vi "Teleop.vi"(10 "Match Info":T3={"Autonomous Elapsed Seconds"=0.0, "TeleOp Elapsed Seconds"=0.0, "Disabled Elapsed Seconds"=0.0, "Visited Autonomous"=FALSE, "Visited TeleOp"=FALSE, "Visited Disabled"=FALSE, "Autonomous Settings"={"Autonomous Style"=enum."Independent", "VI Refnum"=refnum}}, 11 "Call Context":T4) -> ()   [LabVIEW 2020]
doc: "This VI is called for each TeleOp packet received from the DS where the robot is not disabled. It is often used to read from the joysticks and update I/O or to update setpoints for timed control loops. It should complete and return within 20 milliseconds or it may miss DS packets."
uses:
  <vilib>/Rock Robotics/WPI/ThirdParty/Phoenix-LabVIEW/Motor Controller/Controls/CTRE_Phoenix_MotorControl_ControlMode.ctl
  TitanLib/Lib/TitanLib.lvlib
  TitanLib/Lib/Piston Hold.vi
  <vilib>/Rock Robotics/WPI/Solenoid/WPI_SolenoidSetEnum.vi
  <vilib>/Rock Robotics/Network Tables/NT Write Boolean Array.vi
  <vilib>/Rock Robotics/Network Tables/NT Write Numeric Array.vi
  <vilib>/Rock Robotics/WPI/DriverStation/WPI_DriverStationMatch Info.ctl
  <vilib>/Rock Robotics/WPI/DriverStation/WPI_DriverStationDerivedRobotMode.ctl
panel:
  in  "Input 1":bool
  in  "Turret Numeric Value Inputs":T1
  in  "Turret Boolean Value Inputs":T2
  out "Waveform Chart":cluster{"Hood Setpoint":dbl, dbl}(graph)
  in  "ShooterNumeric Value Inputs":T1
  in  "Shooter Boolean Value Inputs":T2
  in  "Climber Numeric Value Inputs":T1={"P"=0.0, "I"=0.0, "D"=0.0, "F"=0.0, "I Zone"=0.0, "Setpoint"=0.0, "Manual Speed Mult"=0.0, "Manual Control Input"=0.0, "Cruise Velocity"=0, "Acceleration"=0, "Percent Deadband"=0.0, "Min Limit"=0.0, "Gear Ratio (x:1)"=15.42}
  in  "error in":errorcluster
  in  "Climber Boolean Value Inputs":T2
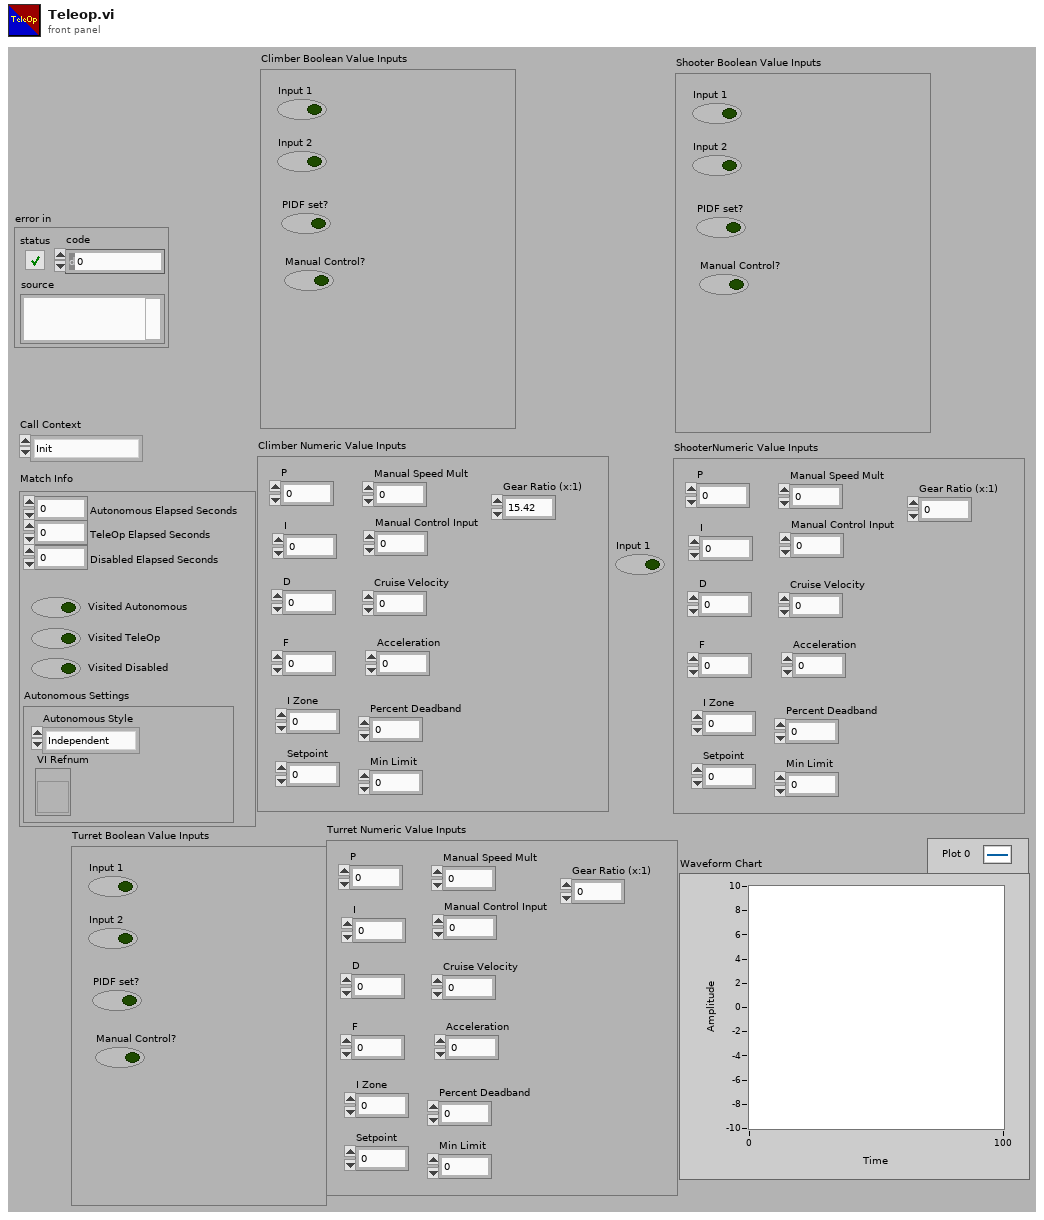
[diagram p1: front panel]
types:
  T1 = cluster{"P":dbl, "I":dbl, "D":dbl, "F":dbl, "I Zone":dbl, "Setpoint":dbl, "Manual Speed Mult":dbl, "Manual Control Input":dbl, "Cruise Velocity":i32, "Acceleration":i32, "Percent Deadband":dbl, "Min Limit":dbl, "Gear Ratio (x:1)":dbl}
  T2 = cluster{"Input 1":bool, "Input 2":bool, "PIDF set?":bool, "Manual Control?":bool}
  T3 = typedef "WPI_DriverStationMatch Info.ctl" = cluster{"Autonomous Elapsed Seconds":dbl, "TeleOp Elapsed Seconds":dbl, "Disabled Elapsed Seconds":dbl, "Visited Autonomous":bool, "Visited TeleOp":bool, "Visited Disabled":bool, "Autonomous Settings":cluster{"Autonomous Style":enum16{"Iterative", "Independent"}, "VI Refnum":refnum<vi>}}
  T4 = typedef "WPI_DriverStationDerivedRobotMode.ctl" = enum16{"Init", "Execute", "Stop"}
  T5 = typedef "CTRE_Phoenix_MotorControl_ControlMode.ctl" = u16
  T6 = cluster{"Climber Up":bool, "Climber Down":bool, "Intake":bool, "Flywheel Power":bool, "Outtake":bool, "Turret Left":bool, "Turret Right":bool}
  T7 = typedef "WPI_JoystickDevRef.ctl" = cluster{"Device":T8}
  T8 = typedef "WPI_JoystickDeviceEnum.ctl" = enum16{"USB 0", "USB 1", "USB 2", "USB 3", "USB 4", "USB 5"}
  T9 = typedef "WPI_MotorControlDeviceRef.ctl" = cluster{"DeviceStatus":errorcluster, "Type":T10, "PWM":cluster{"PWM Channel":T11, "DeadBand":T12}, "CAN":cluster{"Device Number":u8, "SetOutput VI Ref":variant, "GetOutput VI Ref":variant, "Enable VI Ref":variant, "Disable VI Ref":variant, "Data":variant}, "Invert":bool, "DIO PWM":cluster{"PWM \"Enable\" Channel":T11, "DIOChannel":T13, "PWM Rate":dbl}}
  T10 = typedef "WPI_MotorControlType.ctl" = enum16{"PWM", "CAN", "DIO PWM"}
  T11 = typedef "FPGA_DIOPWMChannel.ctl" = enum8{"PWM 0", "PWM 1", "PWM 2", "PWM 3", "PWM 4", "PWM 5", "PWM 6", "PWM 7", "PWM 8", "PWM 9", "PWM MXP 0", "PWM MXP 1", "PWM MXP 2", "PWM MXP 3", "PWM MXP 4", "PWM MXP 5", "PWM MXP 6", "PWM MXP 7", "PWM MXP 8", "PWM MXP 9", "Invalid"}
  T12 = typedef "WPI_PWMDeadband.ctl" = cluster{"Name":string, "maxPositivePwm":i32, "minPositivePwm":i32, "centerPwm":i32, "maxNegativePwm":i32, "minNegativePwm":i32, "angularRange":u16}
  T13 = typedef "FPGA_DIOChannel.ctl" = enum8{"DIO 0", "DIO 1", "DIO 2", "DIO 3", "DIO 4", "DIO 5", "DIO 6", "DIO 7", "DIO 8", "DIO 9", "DIO MXP 0", "DIO MXP 1", "DIO MXP 2", "DIO MXP 3", "DIO MXP 4", "DIO MXP 5", "DIO MXP 6", "DIO MXP 7", "DIO MXP 8", "DIO MXP 9", "DIO MXP 10", "DIO MXP 11", "DIO MXP 12", "DIO MXP 13", "DIO MXP 14", "DIO MXP 15", "SPI Port CS1", "SPI Port CS2", "SPI Port CS3", "SPI Port MISO", "SPI Port MOSI", "Invalid"}
  T14 = typedef "WPI_DigitalInputDevRef.ctl" = cluster{"DevStatus":errorcluster, "DIO Channel":T13}
  T15 = typedef "WPI_SolenoidValue.ctl" = enum16{"Off", "On", "Forward", "Reverse"}
  T16 = typedef "WPI_SolenoidDevRef.ctl" = cluster{"DevStatus":errorcluster, "Pneumatics Control Module":u8, "Forward Solenoid Channel":T17, "Reverse Solenoid Channel":T17}
  T17 = typedef "WPI_SolenoidChannel.ctl" = enum8{"Solenoid 0", "Solenoid 1", "Solenoid 2", "Solenoid 3", "Solenoid 4", "Solenoid 5", "Solenoid 6", "Solenoid 7", "Solenoid 8", "Solenoid 9", "Solenoid 10", "Solenoid 11", "Solenoid 12", "Solenoid 13", "Solenoid 14", "Solenoid 15", "Invalid"}
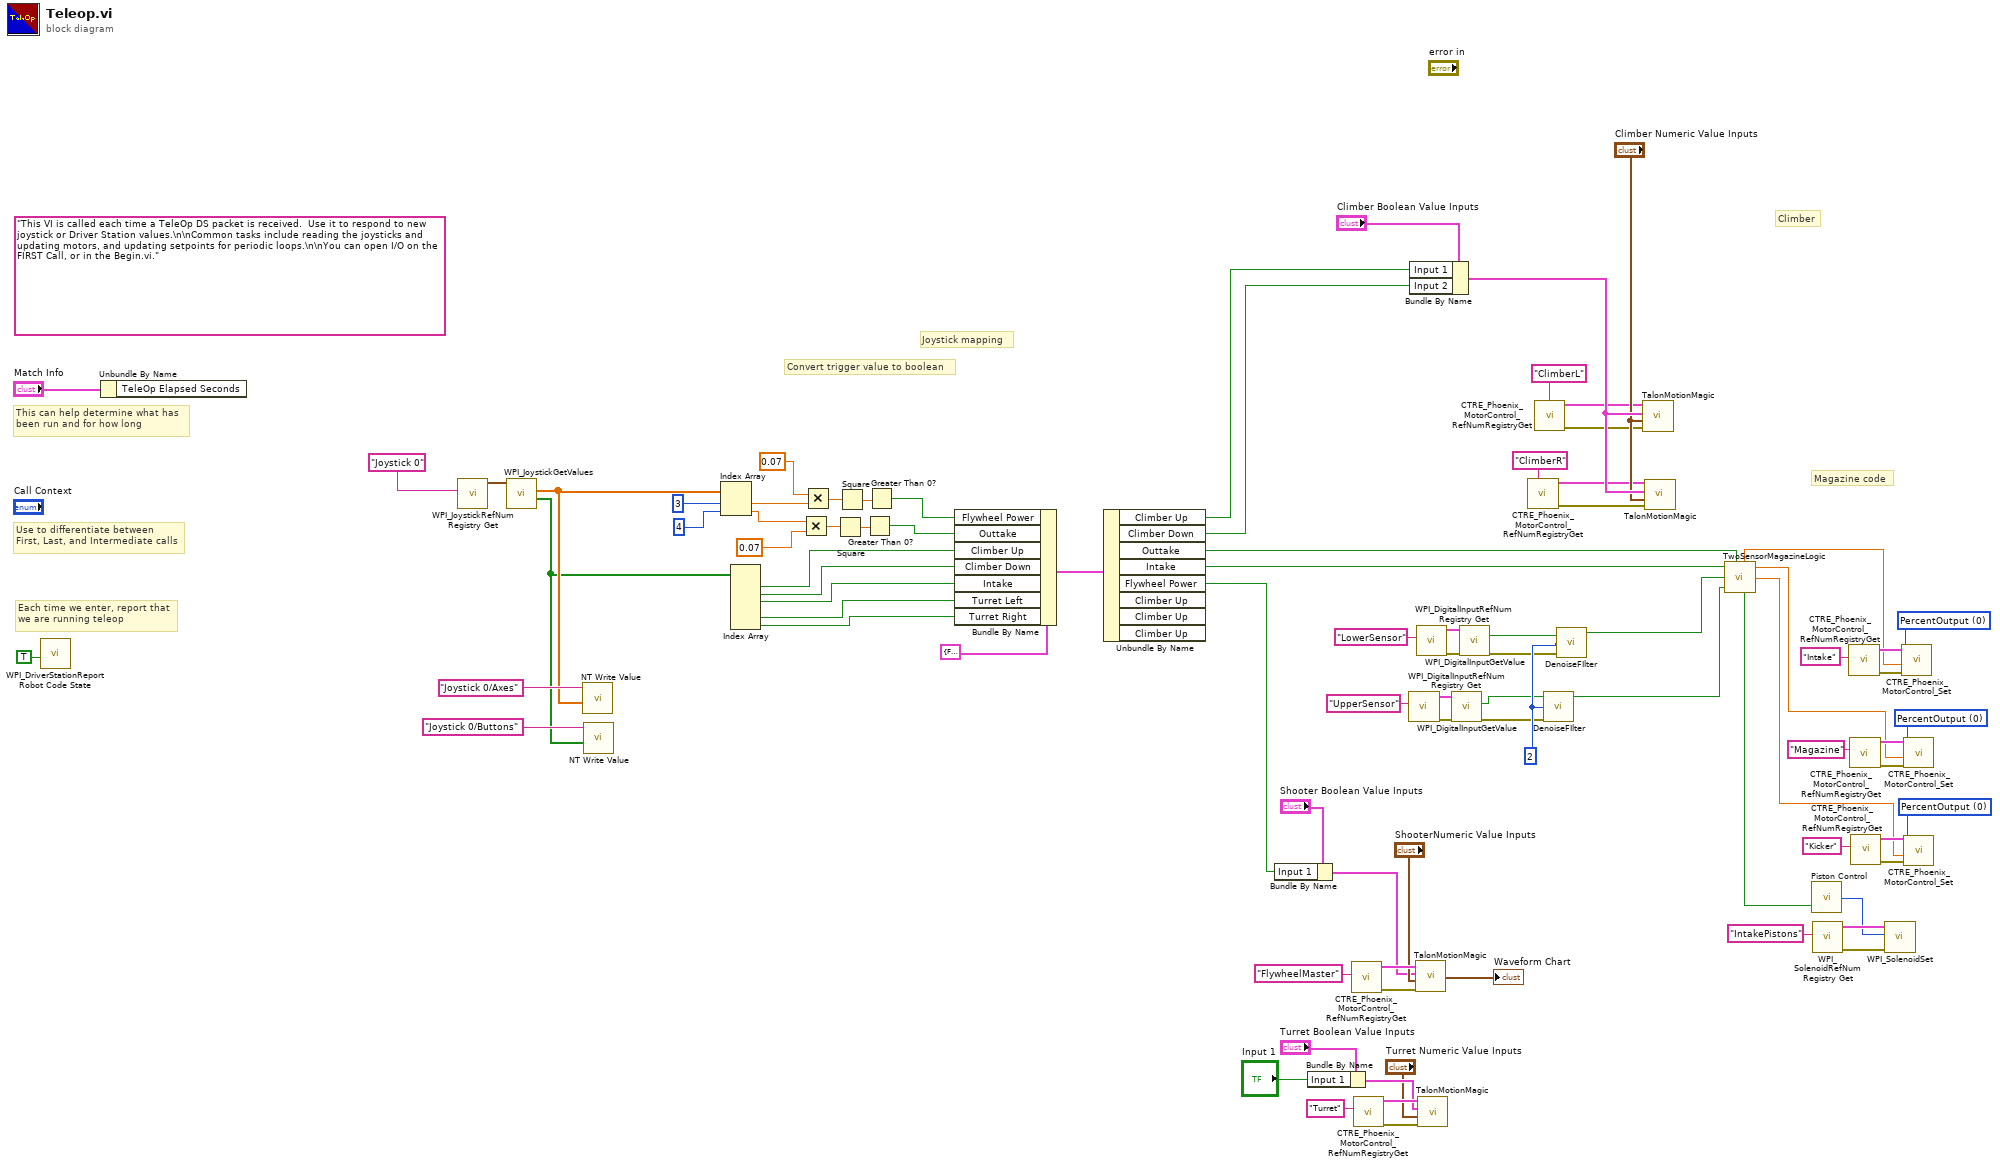
[diagram p0: block diagram]
diagram:
  w24 = T5 0 items=["PercentOutput"=0, "Position"=1, "Velocity"=2, "Current"=3, "Follower"=5, "MotionProfile"=6, "MotionMagic"=7, "MotionProfileArc"=10, "Disabled"=15] ("Control Mode")
  w25 = T5 0 items=["PercentOutput"=0, "Position"=1, "Velocity"=2, "Current"=3, "Follower"=5, "MotionProfile"=6, "MotionMagic"=7, "MotionProfileArc"=10, "Disabled"=15] ("Control Mode")
  w27 = T5 0 items=["PercentOutput"=0, "Position"=1, "Velocity"=2, "Current"=3, "Follower"=5, "MotionProfile"=6, "MotionMagic"=7, "MotionProfileArc"=10, "Disabled"=15] ("Control Mode")
  w45 = 2 ("Filter Level")
  (unwired) "This VI is called each time a TeleOp DS packet is received.  Use it to respond to new joystick or Driver Station values.\n\nCommon tasks include reading the joysticks and updating motors, and updating setpoints for periodic loops.\n\nYou can open I/O on the FIRST Call, or in the Begin.vi."
  # "Convert trigger value to boolean"
  # "Joystick mapping"
  # "Climber"
  # "Magazine code"
  # "Each time we enter, report that\nwe are running teleop"
  # "Use to differentiate between\nFirst, Last, and Intermediate calls"
  # "This can help determine what has\nbeen run and for how long"
  n1 = call <vilib>:"WPI_DriverStationReport Robot Code State.vi"("TeleOp"=TRUE ("Autonomous")) -> ()  [unwired: 10 in, 1 out]
  n2 = Unbundle By Name("Match Info") -> ()  [unwired: 1 out]
  n3 = call <vilib>:"WPI_JoystickRefNum Registry Get.vi"("refnum name"="Joystick 0") -> ("JoystickDevRef"=w86:T7)  [unwired: 1 in, 9 out]
  n4 = call <vilib>:"WPI_JoystickGetValues.vi"("JoystickDevRef"=w86) -> ("Buttons"=w81:bool[], "Axes"=w82:dbl[])  [unwired: 6 in, 3 out]
  n5 = call-poly <vilib>:"NT Write Value.vi"("Numeric Array"=w82, "Name"="Joystick 0/Axes") -> ()  [unwired: 9 in, 1 out]
  n6 = call-poly <vilib>:"NT Write Value.vi"("Boolean Array"=w81, "Name"="Joystick 0/Buttons") -> ()  [unwired: 9 in, 1 out]
  n7 = Index Array(array=w82, index #1=3 ("index"), index #2=4 ("index")) -> (element #1=w77:dbl, element #2=w69:dbl)
  n8 = Index Array(array=w81) -> (element #1=w67:bool, element #2=w66:bool, element #3=w65:bool, element #5=w40:bool, element #6=w41:bool)  [unwired: 6 in, 1 out]
  n9 = Multiply(x=w69, y=0.07 ("x")) -> (x*y=w72:dbl)
  n10 = Multiply(x=0.07, y=w77) -> (x*y=w75:dbl)
  n11 = Square(x=w72) -> (x^2=w71:dbl)
  n12 = Square(x=w75) -> (x^2=w74:dbl)
  n13 = Greater Than 0?(x=w71) -> (x > 0?=w68:bool)
  n14 = Greater Than 0?(x=w74) -> (x > 0?=w73:bool)
  n15 = Bundle By Name(cluster=T6 {"Climber Up"=FALSE, "Climber Down"=FALSE, "Intake"=FALSE, "Flywheel Power"=FALSE, "Outtake"=FALSE, "Turret Left"=FALSE, "Turret Right"=FALSE}, "Flywheel Power"=w73, "Outtake"=w68, "Climber Up"=w67, "Climber Down"=w66, "Intake"=w65, "Turret Left"=w40, "Turret Right"=w41) -> (w64:T6)
  n16 = Unbundle By Name(w64) -> ("Climber Up"=w62:bool, "Climber Down"=w61:bool, "Outtake"=w39:bool, "Intake"=w38:bool, "Flywheel Power"=w12:bool)  [unwired: 3 out]
  n17 = Bundle By Name(cluster="Shooter Boolean Value Inputs", "Input 1"=w12) -> (w13:T2)
  n18 = Bundle By Name(cluster="Turret Boolean Value Inputs", "Input 1"="Input 1") -> (w6:T2)
  n19 = call <vilib>:"CTRE_Phoenix_MotorControl_RefNumRegistryGet.vi"("refnum name"="FlywheelMaster") -> ("error out"=w16:errorcluster, "PhoenixMotorControlDevRef"=w17:T9)  [unwired: 9 in]
  n20 = call <vilib>:"CTRE_Phoenix_MotorControl_RefNumRegistryGet.vi"("refnum name"="Turret") -> ("error out"=w8:errorcluster, "PhoenixMotorControlDevRef"=w9:T9)  [unwired: 9 in]
  n21 = call <vilib>:"WPI_DigitalInputRefNum Registry Get.vi"("refnum name"="UpperSensor") -> ("error out"=w51:errorcluster, "DigitalInputDevRef"=w52:T14)  [unwired: 9 in]
  n22 = Bundle By Name(cluster="Climber Boolean Value Inputs", "Input 1"=w62, "Input 2"=w61) -> (w60:T2)
  n23 = call "TalonMotionMagic.vi"("xMotorControlDevRef"=w17, "Boolean Value Inputs"=w13, "Numeric Value Inputs"="ShooterNumeric Value Inputs", "error in"=w16) -> ("Graph Output"=→"Waveform Chart":cluster{"Hood Setpoint":dbl, dbl})  [unwired: 1 in, 2 out]
  n24 = call <vilib>:"WPI_DigitalInputRefNum Registry Get.vi"("refnum name"="LowerSensor") -> ("error out"=w48:errorcluster, "DigitalInputDevRef"=w47:T14)  [unwired: 9 in]
  n25 = call "TalonMotionMagic.vi"("xMotorControlDevRef"=w9, "Boolean Value Inputs"=w6, "Numeric Value Inputs"="Turret Numeric Value Inputs", "error in"=w8) -> ()  [unwired: 1 in, 3 out]
  n26 = call <vilib>:"WPI_DigitalInputGetValue.vi"("error in (no error)"=w51, "DigitalInputDevRef"=w52) -> ("error out"=w2:errorcluster, "Value"=w44:bool)  [unwired: 7 in, 1 out]
  n27 = call <vilib>:"WPI_DigitalInputGetValue.vi"("error in (no error)"=w48, "DigitalInputDevRef"=w47) -> ("error out"=w3:errorcluster, "Value"=w46:bool)  [unwired: 7 in, 1 out]
  n28 = call <vilib>:"CTRE_Phoenix_MotorControl_RefNumRegistryGet.vi"("refnum name"="ClimberR") -> ("error out"=w54:errorcluster, "PhoenixMotorControlDevRef"=w55:T9)  [unwired: 9 in]
  n29 = call <vilib>:"CTRE_Phoenix_MotorControl_RefNumRegistryGet.vi"("refnum name"="ClimberL") -> ("error out"=w57:errorcluster, "PhoenixMotorControlDevRef"=w58:T9)  [unwired: 9 in]
  n30 = call "DenoiseFIlter.vi"("error in (no error)"=w2, "Filter Level"=w45, "Signal Input"=w44) -> ("Signal Output"=w43:bool)  [unwired: 2 out]
  n31 = call "DenoiseFIlter.vi"("error in (no error)"=w3, "Filter Level"=w45, "Signal Input"=w46) -> ("Signal Output"=w42:bool)  [unwired: 2 out]
  n32 = call "TalonMotionMagic.vi"("xMotorControlDevRef"=w58, "Boolean Value Inputs"=w60, "Numeric Value Inputs"="Climber Numeric Value Inputs", "error in"=w57) -> ()  [unwired: 1 in, 3 out]
  n33 = call "TalonMotionMagic.vi"("xMotorControlDevRef"=w55, "Boolean Value Inputs"=w60, "Numeric Value Inputs"="Climber Numeric Value Inputs", "error in"=w54) -> ()  [unwired: 1 in, 3 out]
  n34 = call "TwoSensorMagazineLogic.vi"("Intake Toggle"=w38, "Outtake Button"=w39, "Intake Side Sensor"=w42, "Outtake Side Sensor"=w43) -> ("Intake Motors"=w28:dbl, "Magazine Motors"=w26:dbl, "Kicker Motors"=w23:dbl, "Intake Pistons"=w19:bool)  [unwired: 1 in, 1 out]
  n35 = call-poly "Piston Control.vi"("Input"=w19) -> ("Output"=w20:T15)  [unwired: 1 in]
  n36 = call <vilib>:"WPI_SolenoidRefNum Registry Get.vi"("refnum name"="IntakePistons") -> ("error out"=w21:errorcluster, "SolenoidDevRef"=w22:T16)  [unwired: 9 in]
  n37 = call <vilib>:"CTRE_Phoenix_MotorControl_RefNumRegistryGet.vi"("refnum name"="Intake") -> ("error out"=w37:errorcluster, "PhoenixMotorControlDevRef"=w36:T9)  [unwired: 9 in]
  n38 = call <vilib>:"CTRE_Phoenix_MotorControl_RefNumRegistryGet.vi"("refnum name"="Magazine") -> ("error out"=w32:errorcluster, "PhoenixMotorControlDevRef"=w33:T9)  [unwired: 9 in]
  n39 = call <vilib>:"CTRE_Phoenix_MotorControl_RefNumRegistryGet.vi"("refnum name"="Kicker") -> ("error out"=w35:errorcluster, "PhoenixMotorControlDevRef"=w34:T9)  [unwired: 9 in]
  n40 = call-poly <vilib>:"WPI_SolenoidSet.vi"("error in (no error)"=w21, "Value"=w20, "SolenoidDevRef"=w22) -> ()  [unwired: 7 in, 2 out]
  n41 = call <vilib>:"CTRE_Phoenix_MotorControl_Set.vi"("error in (no error)"=w37, "Output"=w28, "Control Mode"=w27, "PhoenixMotorControlDevRef"=w36) -> ()  [unwired: 6 in, 2 out]
  n42 = call <vilib>:"CTRE_Phoenix_MotorControl_Set.vi"("error in (no error)"=w32, "Output"=w26, "Control Mode"=w25, "PhoenixMotorControlDevRef"=w33) -> ()  [unwired: 6 in, 2 out]
  n43 = call <vilib>:"CTRE_Phoenix_MotorControl_Set.vi"("error in (no error)"=w35, "Output"=w23, "Control Mode"=w24, "PhoenixMotorControlDevRef"=w34) -> ()  [unwired: 6 in, 2 out]
